vi "Read State.vi"(7 "timeout in ms (-1)":i32=-1, 8 "error in (no error)":errorcluster, 9 "Return Boolean Array? (F)":bool, 11 "Storage Line in":refnum<class "Storage Line.lvclass">) -> (0 "error out":errorcluster, 1 "Boolean array":bool[](array[boolean]), 2 "State":u16, 3 "Storage Line out":refnum<class "Storage Line.lvclass">, 4 "Line StateQ":refnum<queue>)   [LabVIEW 2015, in "cRIO-Carbondioxide.lvlib" / "CO2-Actor.lvlib" / "Storage Line.lvclass"]
uses:
  Storage Line.lvclass
  Storage Line.lvclass/Storage Line.ctl
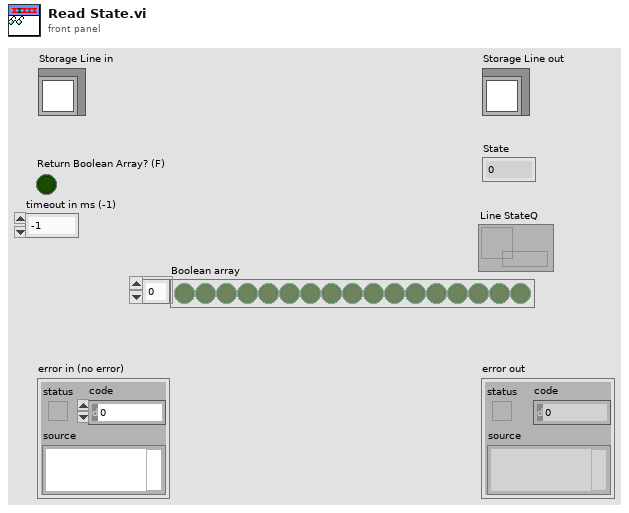
[diagram p1: front panel]
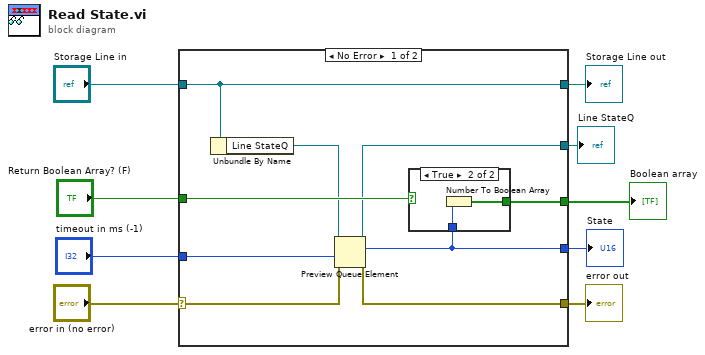
[diagram p0: block diagram]
diagram:
  n1 = case shown="No Error" "error in (no error)" {
    selector: "error in (no error)" -> [w13 w21]
    tunnel: [w12 w21] -> w8
    tunnel: [w18 w22] -> w6
    tunnel: "Storage Line in" -> [w18 w22]
    tunnel: [w14 _] -> w2
    tunnel: [w17 _] -> w5
    tunnel: "Return Boolean Array? (F)" -> [w16 _]
    tunnel: [w11 _] -> w3
    tunnel: "timeout in ms (-1)" -> [w10 _]
    frame No Error {
      n2 = Unbundle By Name(w18) -> ("Line StateQ"=w15:refnum<queue>)
      n3 = Preview Queue Element(queue=w15, timeout in ms (-1)=w10, error in (no error)=w13) -> (queue out=w14:refnum<queue>, element=w11:u16, error out=w12:errorcluster)  [unwired: 1 out]
      n4 = case shown="True" w16 {
        tunnel: [_ w20] -> w17
        tunnel: w11 -> [_ w19]
        frame False {
        }
        frame True {
          n5 = Number To Boolean Array(number=w19) -> (Boolean array=w20:bool[])
        }
      }
    }
    frame Error {
    }
  }
  "error out" <- w8
  "Storage Line out" <- w6
  "State" <- w3
  "Boolean array" <- w5
  "Line StateQ" <- w2
